vi "Process.vi"(8 "error in":errorcluster, 11 "Plugin in":refnum<class "Adjust Block Size.lvclass">) -> (0 "error out":errorcluster, 3 "Plugin out":refnum<class "Adjust Block Size.lvclass">)   [LabVIEW 2024, in "Adjust Block Size.lvlib" / "Adjust Block Size.lvclass"]
uses:
  Adjust Block Size.lvclass
  Adjust Block Size.lvclass/Adjust Block Size.ctl
  <vilib>/addons/_NISVFA/_Shared subVIs/Data Objects/Data/Data.lvclass/Data.ctl
  <vilib>/addons/_NISVFA/_Shared subVIs/Data Objects/Data/Read Data Increment.vi
  <vilib>/addons/_NISVFA/_Shared subVIs/Data Objects/Data/Read Data Attributes.vi
  <vilib>/addons/_NISVFA/_Shared subVIs/Data Objects/subVIs/Get Data Sample Interval (dt).vi
  <vilib>/addons/_NISVFA/_Shared subVIs/Common/sv_Get NI Property Name String.vi
  <vilib>/addons/_NISVFA/_Shared subVIs/Data Objects/Waveforms (DBL)/Waveforms (N Ch).lvclass
  <vilib>/addons/_NISVFA/_Shared subVIs/Data Objects/Waveforms (DBL)/SV Read Next Continuous Data.vi
  <vilib>/FlexLogger/SDK/PluginSDK.lvlibp/PEFClasses/SDK/Plugin/DataHelpers/Write 1D Wfm (DBL)_v2.vi
  <vilib>/FlexLogger/SDK/PluginSDK.lvlibp/PEFClasses/SDK/Plugin/Plugin.lvclass
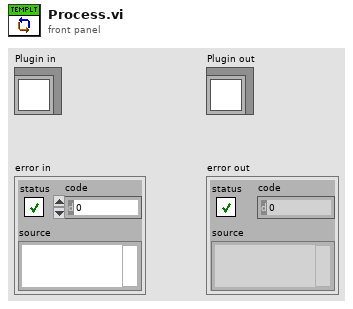
[diagram p1: front panel]
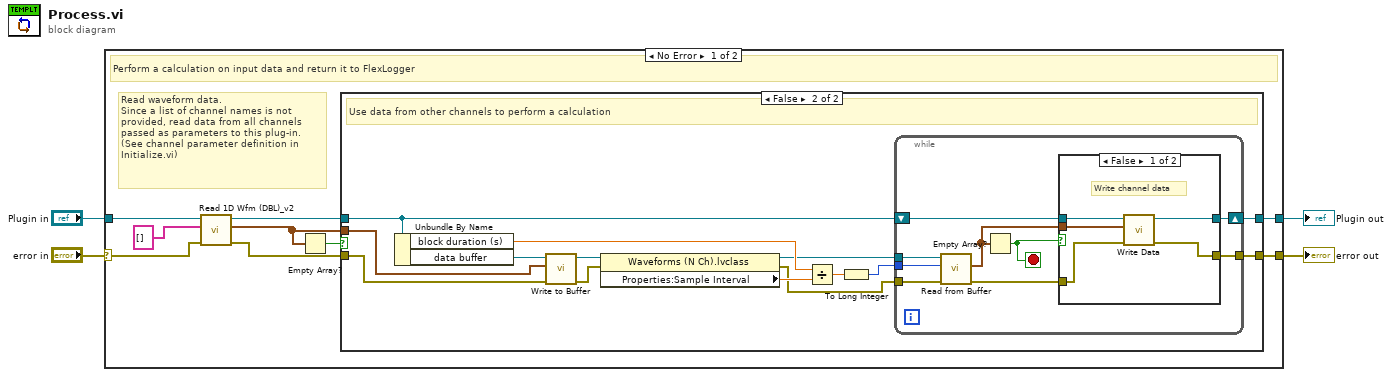
[diagram p0: block diagram]
diagram:
  n1 = case shown="No Error" "error in" {
    selector: "error in" -> [w12 w45]
    tunnel: [w10 w46] -> w1
    tunnel: "Plugin in" -> [w13 w46]
    tunnel: [w11 w45] -> w2
    frame No Error {
      # "Read waveform data.\nSince a list of channel names is not provided, read data from all channels passed as parameters to this plug-in.\n(See channel parameter definition in Initialize.vi)"
      # "Perform a calculation on input data and return it to FlexLogger"
      n2 = call <vilib>:"Read 1D Wfm (DBL)_v2.vi"("error in (no error)"=w12, "Unique Identifers (empty = all)"=string[] [] ("Unique Channel Identifers (empty = all)"), "Plugin in"=w13) -> ("error out"=w8:errorcluster, "Data"=w6:waveform(dbl)[], "Plugin out"=w9:refnum<class "Adjust Block Size.lvclass">)  [unwired: 5 in, 1 out]
      n3 = Empty Array?(array=w6) -> (empty?=w5:bool)
      n4 = case shown="False" w5 {
        tunnel: w6 -> [_ w24]
        tunnel: [w14 w29] -> w11
        tunnel: [w15 w28] -> w10
        tunnel: w9 -> [w15 w27]
        tunnel: w8 -> [w14 w26]
        frame True {
          # "No channels sending data to the plugin"
        }
        frame False {
          # "Use data from other channels to perform a calculation"
          n5 = Unbundle By Name(w27) -> ("block duration (s)"=w21:dbl, "data buffer"=w25:refnum<data-value>)
          n6 = call <vilib>:"Write to Buffer.vi"("error in (no error)"=w26, "waveforms"=w24, "buffer"=w25) -> ("error out"=w22:errorcluster, "buffer out"=w23:refnum<data-value>)  [unwired: 6 in, 1 out]
          n7 = property class="Waveforms (N Ch).lvclass"(reference=w23, error in=w22) -> (reference out=w17:refnum<data-value>, error out=w16:errorcluster, "Properties:Sample Interval"=w20:dbl)
          n8 = Divide(x=w21, y=w20) -> (x/y=w19:dbl)
          n9 = To Long Integer(number=w19) -> (32bit integer=w18:i32)
          n10 = while {
            tunnel: [w38] -> w29
            tunnel: w18 -> [w35]
            tunnel: w17 -> [w34]
            tunnel: w16 -> [w33]
            shift-right: [w37] -> w28
            shift-left: w27 -> [w36]
            stop <- w30 stop-if-true
            n11 = call-poly <vilib>:"Read from Buffer.vi"("error in (no error)"=w33, "block length (-1 = all)"=w35, "buffer"=w34) -> ("error out"=w31:errorcluster, "waveforms subset"=w32:waveform(dbl)[])  [unwired: 5 in, 2 out]
            n12 = Empty Array?(array=w32) -> (empty?=w30:bool)
            n13 = case shown="False" w30 {
              tunnel: [w43 _] -> w38
              tunnel: [w42 w44] -> w37
              tunnel: w36 -> [w41 w44]
              tunnel: w32 -> [w40 _]
              tunnel: w31 -> [w39 _]
              frame False {
                # "Write channel data"
                n14 = call-poly <vilib>:"Write Data.vi"("error in (no error)"=w39, "Data"=w40, "Plugin in"=w41) -> ("error out"=w43:errorcluster, "Plugin out"=w42:refnum<class "Adjust Block Size.lvclass">)  [unwired: 7 in]
              }
              frame True {
              }
            }
          }
        }
      }
    }
    frame Error {
    }
  }
  "error out" <- w2
  "Plugin out" <- w1
